vi "define error position.vi"(8 "Position":i32, 11 "error in (no error)":errorcluster) -> (0 "first error position":i32, 3 "error out":errorcluster)   [LabVIEW 2009, in "MoAgSy.lvlib"]
uses:
  MoAgSy.lvlib
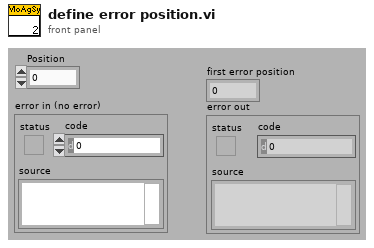
[diagram p1: front panel]
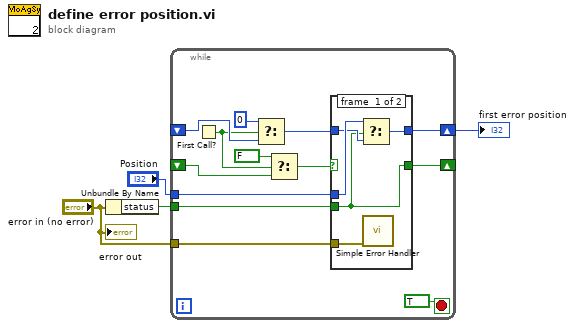
[diagram p0: block diagram]
diagram:
  n1 = Unbundle By Name("error in (no error)") -> ("status"=w4:bool)
  n2 = while {
    tunnel: w4 -> [w17]
    shift-right: [w15] -> w2
    shift-left: _ -> [w13]
    shift-right: [w14] -> _
    shift-left: _ -> [w8]
    tunnel: "Position" -> [w16]
    tunnel: "error in (no error)" -> [w5]
    stop <- TRUE stop-if-true
    n3 = First Call?() -> (First Call?: T/F=w7:bool)
    n4 = Select(t=0, s=w7, f=w13) -> (s? t:f=w11:i32)
    n5 = Select(t=FALSE, s=w7, f=w8) -> (s? t:f=w9:bool)
    n6 = case shown="False" w9 {
      selector: w9 -> [_ w23]
      tunnel: w17 -> [w19 _]
      tunnel: w16 -> [w22 _]
      tunnel: [w21 w24] -> w15
      tunnel: w11 -> [w20 w24]
      tunnel: [w19 w23] -> w14
      tunnel: w5 -> [w18 _]
      frame #0 {
        n7 = Select(t=w22, s=w19, f=w20) -> (s? t:f=w21:i32)
        n8 = call <vilib>:"Simple Error Handler.vi"("error in (no error)"=w18) -> ()  [unwired: 4 in, 5 out]
      }
      frame #1 {
      }
    }
  }
  "first error position" <- w2
  "error out" <- "error in (no error)"
